vi "Save Variant to JSON File.vi"   [LabVIEW 2017, in "Variant JSON API.lvlib"]
doc: "Saves a JSON instance's data to the given file."
uses:
  Variant JSON API.lvlib
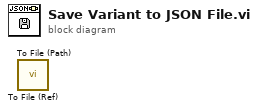
[diagram p0: block diagram]
diagram:
  n1 = call "To File (Ref).vi"() -> ()  [unwired: 10 in, 2 out]
  n2 = call "To File (Path).vi"() -> ()  [unwired: 10 in, 2 out]
